vi "tagDB_Value_Template_RegExp.vi"(8 "error in (no error)":errorcluster, 9 "Type":variant, 10 "RegExp":string, 11 "DB Ref":T1) -> (0 "error out":errorcluster, 1 "names":string[](array[string]), 2 "value":variant[](array[variant]), 3 "DB Ref(dup)":T1)   [LabVIEW 2014, in "TagDB(dev).lvlib"]
doc: "[Covers: REQ_TAGDB_TEMPLATE_VALUE_REGEXP]"
uses:
  tagDB_Def.ctl
  Error/_[error50001]Can't Found Value.vi
  Private/_Cast TagDB Ref to DVR.vi
  _global/URL/TRIM-BOTH-SPACE.vi
  Error/_[error50000]Invalid DB REF.vi
  TagDB(dev).lvlib
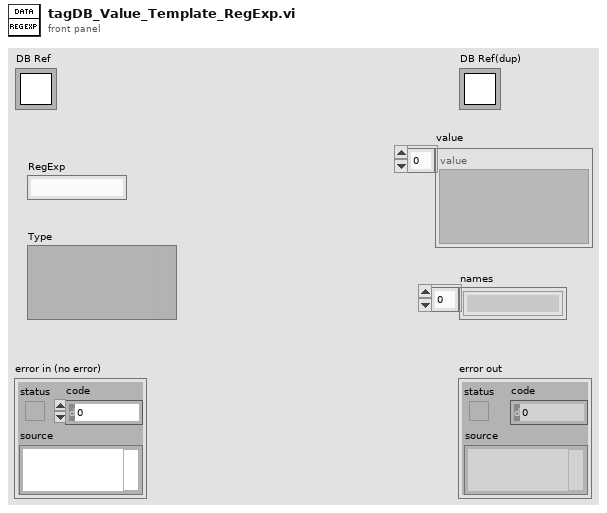
[diagram p1: front panel]
types:
  T1 = typedef "TagDB(dev).lvlib/tagDB_Def.ctl" = refnum<k1>
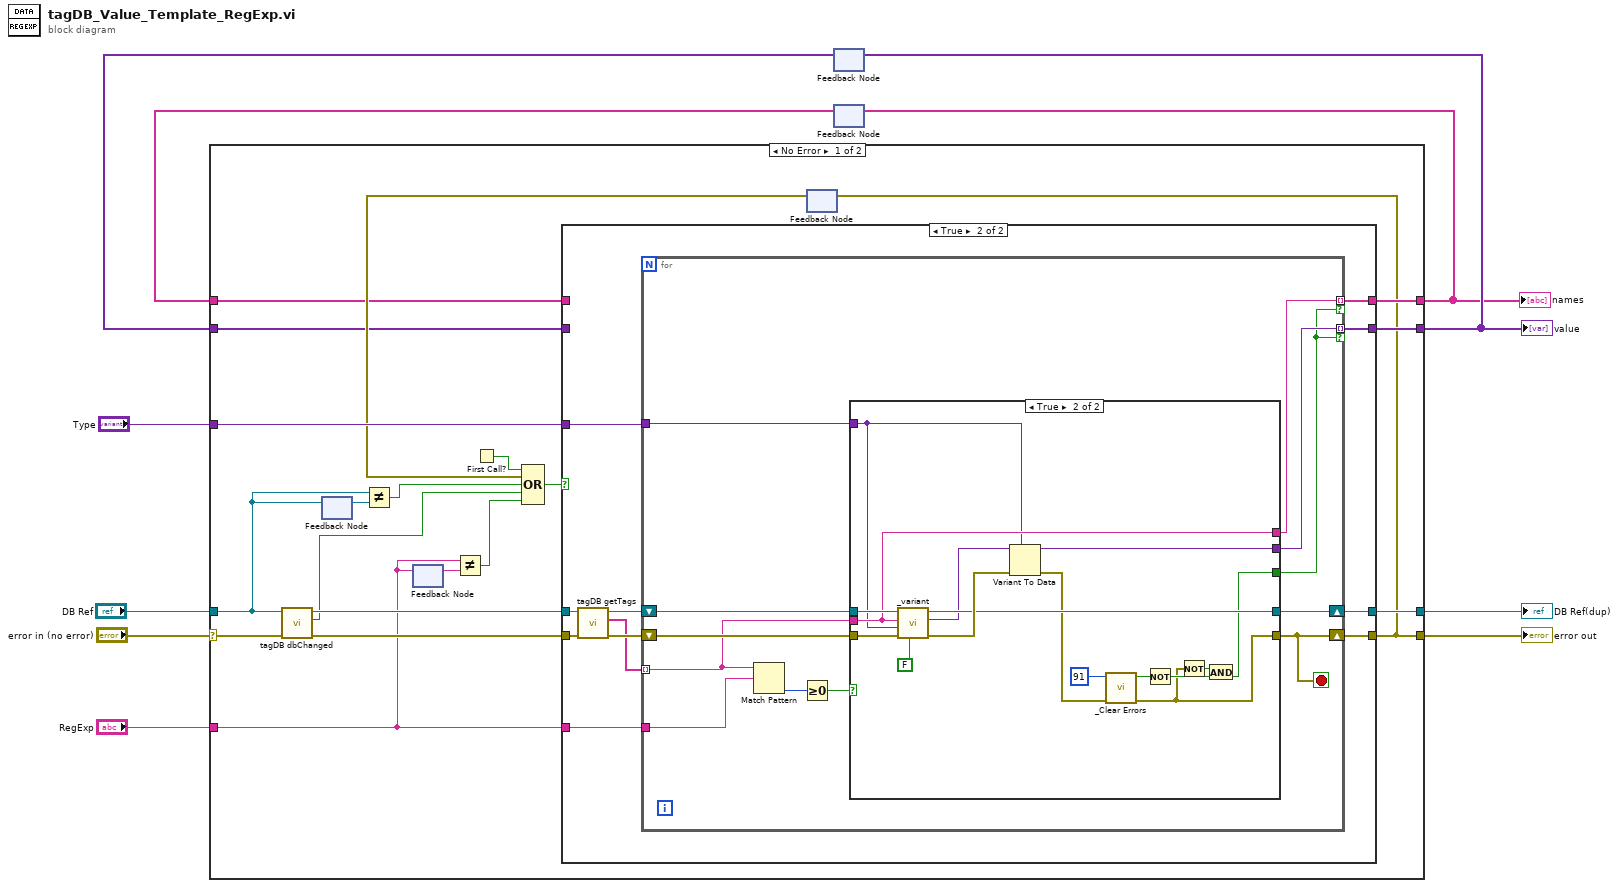
[diagram p0: block diagram]
diagram:
  n1 = feedback #1() -> (w3:variant[])  [unwired: 1 in]
  n2 = feedback #2() -> (w1:string[])  [unwired: 1 in]
  n3 = case shown="No Error" "error in (no error)" {
    selector: "error in (no error)" -> [w25 w80]
    tunnel: [w15 w80] -> w9
    tunnel: [w30 w79] -> w7
    tunnel: "DB Ref" -> [w18 w79]
    tunnel: "RegExp" -> [w16 _]
    tunnel: "Type" -> [w28 _]
    tunnel: [w29 w78] -> w4
    tunnel: [w27 w77] -> w2
    tunnel: w3 -> [w12 w78]
    tunnel: w1 -> [w11 w77]
    frame No Error {
      n4 = call "tagDB dbChanged.vi"("error in (no error)"=w25, "DB Ref"=w18) -> ("error in (no error) (dup)"=w24:errorcluster, "changed?"=w17:bool, "DB Ref (dup)"=w26:T1)  [unwired: 7 in]
      n5 = feedback #3() -> (w22:T1)  [unwired: 1 in]
      n6 = feedback-in #3(w18) -> ()
      n7 = Not Equal?(x=w18, y=w22) -> (x != y?=w20:bool)
      n8 = feedback #4() -> (w21:string)  [unwired: 1 in]
      n9 = feedback-in #4(w16) -> ()
      n10 = Not Equal?(x=w16, y=w21) -> (x != y?=w19:bool)
      n11 = First Call?() -> (First Call?: T/F=w23:bool)
      n12 = feedback #5() -> (w14:errorcluster)  [unwired: 1 in]
      n13 = Compound Arithmetic op=OR(w23, w14, w20, w17, w19) -> (w13:bool)
      n14 = case shown="True" w13 {
        tunnel: [w32 w45] -> w30
        tunnel: [w34 w44] -> w29
        tunnel: w28 -> [_ w43]
        tunnel: [w33 w39] -> w27
        tunnel: w26 -> [w32 w38]
        tunnel: w24 -> [w31 w37]
        tunnel: w16 -> [_ w36]
        tunnel: [w31 w35] -> w15
        tunnel: w12 -> [w34 _]
        tunnel: w11 -> [w33 _]
        frame False {
        }
        frame True {
          n15 = call "tagDB getTags.vi"("error in (no error)"=w37, "DB Ref in"=w38) -> ("error out"=w41:errorcluster, "DB items"=w40:string[], "DB Ref out"=w42:T1)  [unwired: 7 in]
          n16 = for {
            tunnel: w36 -> [w52]
            shift-right: [w57] -> w45
            shift-left: w42 -> [w55]
            shift-right: [w50] -> w35
            shift-left: w41 -> [w54]
            tunnel: w43 -> [w53]
            tunnel: [w56] -> w44 mode=indexing if=w48
            tunnel: w40 -> [w47] mode=indexing
            tunnel: [w49] -> w39 mode=indexing if=w48
            stop <- w50 stop-if-true
            n17 = Match Pattern(string=w47, regular expression=w52) -> (offset past match=w46:i32)  [unwired: 1 in, 3 out]
            n18 = Greater Or Equal To 0?(x=w46) -> (x >= 0?=w51:bool)
            n19 = case shown="True" w51 {
              tunnel: [w59 w65] -> w50
              tunnel: [w60 w75] -> w57
              tunnel: [w58 w73] -> w56
              tunnel: w55 -> [w60 w72]
              tunnel: w54 -> [w59 w71]
              tunnel: w53 -> [w58 w62]
              tunnel: [_ w66] -> w48
              tunnel: [_ w63] -> w49
              tunnel: w47 -> [_ w63]
              frame False {
              }
              frame True {
                n20 = call "_variant.vi"("Add wih NonExist?"=FALSE, "error in (no error)"=w71, "default value (empty variant)"=w62, "name"=w63, "DB Ref"=w72) -> ("error out"=w76:errorcluster, "value"=w74:variant, "DB Ref (dup)"=w75:T1)  [unwired: 4 in]
                n21 = Variant To Data(error in=w76, type=w62, Variant=w74) -> (data=w73:variant, error out=w70:errorcluster)
                n22 = call "_Clear Errors.vi"("error in (no error)"=w70, "specific error code to clear (0: all)"=91) -> ("error out"=w65:errorcluster, "specific error cleared?"=w68:bool)  [unwired: 4 in]
                n23 = Not(x=w68) -> (.not. x?=w67:bool)
                n24 = Not(x=w65) -> (.not. x?=w64:bool)
                n25 = And(x=w64, y=w67) -> (x .and. y?=w66:bool)
              }
            }
          }
        }
      }
      n26 = feedback-in #5(w15) -> ()
    }
    frame Error {
    }
  }
  "error out" <- w9
  "DB Ref(dup)" <- w7
  "value" <- w4
  "names" <- w2
  n27 = feedback-in #1(w4) -> ()
  n28 = feedback-in #2(w2) -> ()
